vi "Teleop-Sub-ArmControls.vi"(0 "Servo Refnum Name":string, 1 "Move Arm?":bool, 2 "Go Up?":bool, 3 "Scale Factor":dbl) -> (7 "Position":dbl)   [LabVIEW 2016]
doc: "The TeleOp arm control VI controls the robot arm. It takes in the following parameters:\n - State: The control state - Boolean\n - Up - Boolean\n - Down - Boolean\n - Scale factor : DBL - How fast the arm moves (from 0.001 to 0.1)\n\nOptionally it outputs the position of the arm."
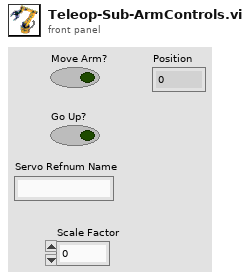
[diagram p1: front panel]
types:
  T1 = typedef "WPI_ServoDeviceRef.ctl" = cluster{"DeviceStatus":errorcluster, "PWM Channel":T2, "DeadBand":T3}
  T2 = typedef "FPGA_DIOPWMChannel.ctl" = enum8{"PWM 0", "PWM 1", "PWM 2", "PWM 3", "PWM 4", "PWM 5", "PWM 6", "PWM 7", "PWM 8", "PWM 9", "PWM MXP 0", "PWM MXP 1", "PWM MXP 2", "PWM MXP 3", "PWM MXP 4", "PWM MXP 5", "PWM MXP 6", "PWM MXP 7", "PWM MXP 8", "PWM MXP 9", "Invalid"}
  T3 = typedef "WPI_PWMDeadband.ctl" = cluster{"Name":string, "maxPositivePwm":i32, "minPositivePwm":i32, "centerPwm":i32, "maxNegativePwm":i32, "minNegativePwm":i32, "angularRange":u16}
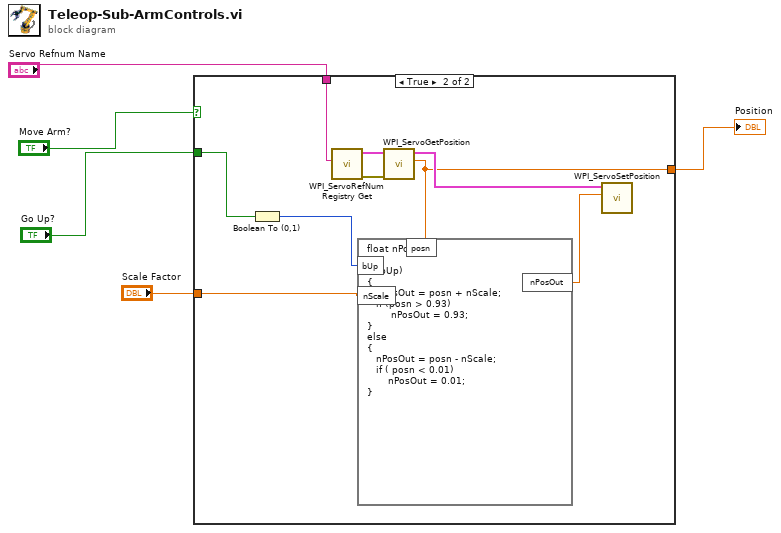
[diagram p0: block diagram]
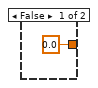
[diagram p2: hidden frame]
diagram:
  n1 = case shown="True" "Move Arm?" {
    tunnel: "Go Up?" -> [_ w12]
    tunnel: "Scale Factor" -> [_ w9]
    tunnel: [0.0 ("Position") w8] -> w5
    tunnel: "Servo Refnum Name" -> [_ w7]
    frame False {
    }
    frame True {
      n2 = Boolean To (0,1)(Boolean=w12) -> (0, 1=w11:i16)
      n3 = call <vilib>:"WPI_ServoRefNum Registry Get.vi"("refnum name"=w7) -> ("error out"=w15:errorcluster, "ServoDeviceRef"=w14:T1)  [unwired: 9 in]
      n4 = call <vilib>:"WPI_ServoGetPosition.vi"("error in (no error)"=w15, "ServoDeviceRef"=w14) -> ("Position"=w8:dbl, "ServoDeviceRef"=w13:T1)  [unwired: 7 in, 1 out]
      n5 = formula code="float nPosOut;\n\nif (bUp) \n{\n   nPosOut = posn + nScale;\n   if (posn > 0.93) \n        nPosOut = 0.93; \n}\nelse\n{\n   nPosOut = posn - nScale;\n   if ( posn < 0.01)\n       nPosOut = 0.01;\n}"("posn"=w8, "bUp"=w11, "nScale"=w9) -> ("nPosOut"=w10:dbl)
      n6 = call <vilib>:"WPI_ServoSetPosition.vi"("Position"=w10, "ServoDeviceRef"=w13) -> ()  [unwired: 8 in, 2 out]
    }
  }
  "Position" <- w5
